vi "User Interface.vi"(8 "error in":errorcluster, 11 "User Interface in":refnum<class "User Interface.lvclass">=refnum) -> (0 "error out":errorcluster, 3 "User Interface out":refnum<class "User Interface.lvclass">)   [LabVIEW 2020, in "RDMA.lvlib" / "RDMA Transfer Tx User Interface.lvclass"]
uses:
  RDMA Transfer Tx User Interface.lvclass
  Configuration/Tx Transfer/RDMA Transfer Tx Configuration.lvclass
  DSF Core.lvlibp/Classes/User Interface/User Interface.lvclass
panel:
  in  "Local Port":u16
  in  "Local Address":string
  in  "Destination Address":string
  in  "Destination Port":u16
  # "RDMA Plugin Settings"
  # "* The address fields must be in IP dot notation. \n   Example: 10.0.53.23"
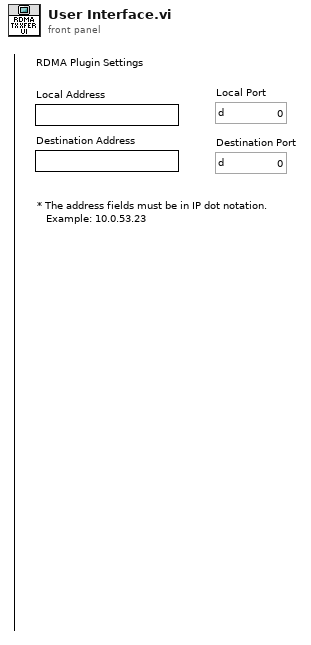
[diagram p1: front panel]
types:
  T1 = typedef "RDMA.lvlib/RDMA Transfer Tx Configuration.lvclass/Tx Transfer Settings.ctl" = cluster{"local address":u32, "local port":u16, "destination address":u32, "destination port":u16}
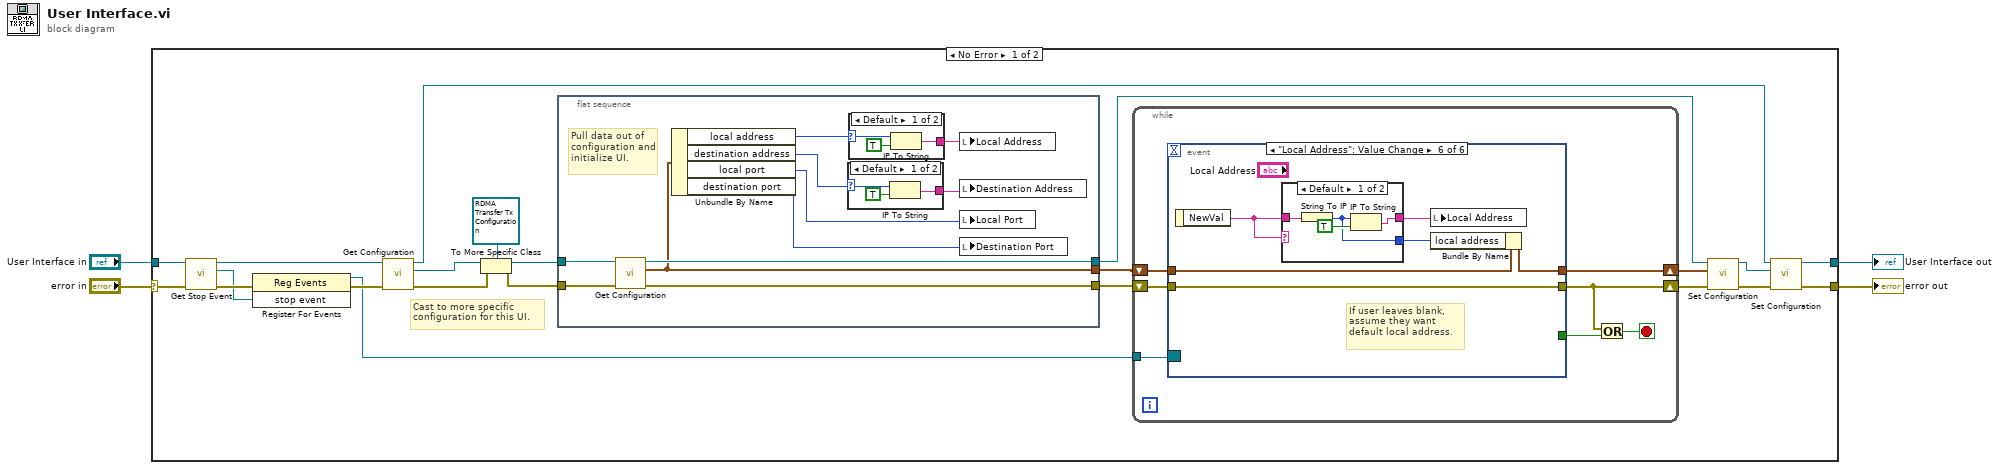
[diagram p0: block diagram]
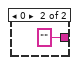
[diagram p2: hidden frame]
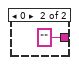
[diagram p3: hidden frame]
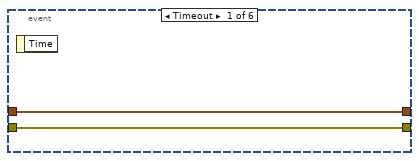
[diagram p4: hidden frame]
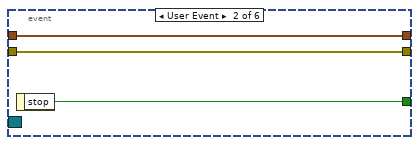
[diagram p5: hidden frame]
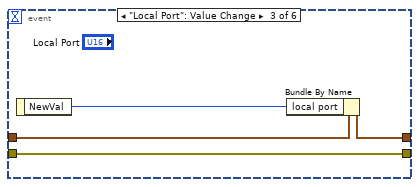
[diagram p6: hidden frame]
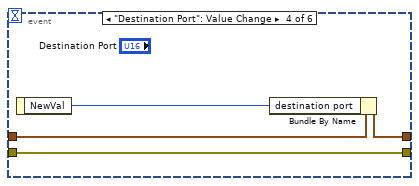
[diagram p7: hidden frame]
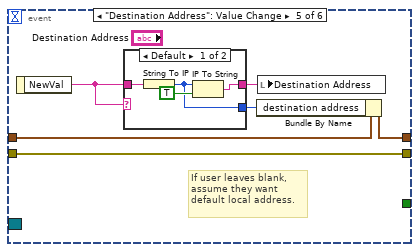
[diagram p8: hidden frame]
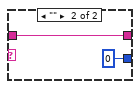
[diagram p9: hidden frame]
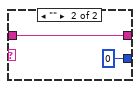
[diagram p10: hidden frame]
diagram:
  n1 = case shown="No Error" "error in" {
    selector: "error in" -> [w26 w91]
    tunnel: [w17 w91] -> w4
    tunnel: "User Interface in" -> [w25 w90]
    tunnel: [w16 w90] -> w1
    frame No Error {
      # "Cast to more specific configuration for this UI."
      n2 = call "Get Stop Event.vi"("error in (no error)"=w26, "User Interface in"=w25) -> ("error out"=w24:errorcluster, "stop event"=w23:refnum<user-event>, "User Interface out"=w22:refnum<class "User Interface.lvclass">)  [unwired: 7 in]
      n3 = register-events(error in=w24, w23) -> (reference out=w20:refnum<event-registration>, error out=w21:errorcluster)  [unwired: 1 in]
      n4 = call "Get Configuration.vi"("error in (no error)"=w21, "User Interface in"=w22) -> ("error out"=w19:errorcluster, "configuration"=w18:refnum<class "Configuration.lvclass">, "User Interface out"=w15:refnum<class "User Interface.lvclass">)  [unwired: 7 in]
      n5 = To More Specific Class(target class=refnum<class "RDMA Transfer Tx Configuration.lvclass"> refnum ("DSF Core.lvlib:UDP Transfer Tx Configuration.lvclass"), reference=w18, error in=w19) -> (specific class reference=w9:refnum<class "RDMA Transfer Tx Configuration.lvclass">, error out=w8:errorcluster)
      n6 = flat-sequence {
        tunnel: [w35] -> w5
        tunnel: w8 -> [w37]
        tunnel: w9 -> [w36]
        tunnel: [w33] -> w7
        tunnel: [w32] -> w6
        frame #0 {
          # "Pull data out of configuration and initialize UI."
          n7 = call "Get Configuration.vi"("error in"=w37, "RDMA Transfer Tx Configuration in"=w36) -> ("error out"=w35:errorcluster, "transfer settings"=w32:T1, "RDMA Transfer Tx Configuration out"=w33:refnum<class "RDMA Transfer Tx Configuration.lvclass">)  [unwired: 7 in]
          n8 = Unbundle By Name(w32) -> ("local address"=w31:u32, "destination address"=w30:u32, "local port"=w28:u16, "destination port"=w27:u16)
          n9 = case shown="Default" w30 {
            selector: w30 -> [w38 _]
            tunnel: [w40 "" ("name")] -> w29
            frame Default {
              n10 = IP To String(1:TRUE ("dot notation? (F)"), 2:w38) -> (0:w40:string)
            }
            frame 0 {
            }
          }
          n11 = case shown="Default" w31 {
            selector: w31 -> [w42 _]
            tunnel: [w44 "" ("name")] -> w34
            frame Default {
              n12 = IP To String(1:TRUE ("dot notation? (F)"), 2:w42) -> (0:w44:string)
            }
            frame 0 {
            }
          }
          n13 = local write "Local Address"(w34) -> ()
          n14 = local write "Destination Address"(w29) -> ()
          n15 = local write "Local Port"(w28) -> ()
          n16 = local write "Destination Port"(w27) -> ()
        }
      }
      n17 = while {
        tunnel: w20 -> [w49]
        shift-right: [w47] -> w13
        shift-left: w5 -> [w50]
        shift-right: [w46] -> w11
        shift-left: w6 -> [w51]
        stop <- w52 stop-if-true
        n18 = event shown="[5] \"Local Address\": Value Change" {
          selector: w49 -> [_ _ _ _ _ _]
          dyn-events: _ -> [_ _ _ _ _ _]
          timeout: _ -> [_ _ _ _ _ _]
          tunnel: [_ w56 _ _ _ _] -> w48
          tunnel: w50 -> [w54 w57 w61 w65 w68 w80]
          tunnel: [w54 w57 w61 w65 w68 w80] -> w47
          tunnel: w51 -> [w53 w55 w60 w64 w69 w81]
          tunnel: [w53 w55 w59 w63 w71 w83] -> w46
          event Timeout {
            n19 = event-data() -> ()  [unwired: 1 in, 1 out]
          }
          event User Event {
            n20 = event-data() -> ("stop"=w56:bool)  [unwired: 1 in]
          }
          event "Local Port": Value Change {
            n21 = event-data() -> ("NewVal"=w58:u16)  [unwired: 1 in]
            n22 = Bundle By Name(cluster=w60, "local port"=w58) -> (w59:T1)
          }
          event "Destination Port": Value Change {
            n23 = event-data() -> ("NewVal"=w62:u16)  [unwired: 1 in]
            n24 = Bundle By Name(cluster=w64, "destination port"=w62) -> (w63:T1)
          }
          event "Destination Address": Value Change {
            # "If user leaves blank, assume they want default local address."
            n25 = event-data() -> ("NewVal"=w66:string)  [unwired: 1 in]
            n26 = case shown="Default" w66 {
              tunnel: [w75 w76] -> w70
              tunnel: w66 -> [w74 w76]
              tunnel: [w72 u32 0] -> w67
              frame Default {
                n27 = String To IP(1:w74) -> (0:w72:u32)
                n28 = IP To String(1:TRUE ("dot notation? (F)"), 2:w72) -> (0:w75:string)
              }
              frame "" {
              }
            }
            n29 = Bundle By Name(cluster=w69, "destination address"=w67) -> (w71:T1)
            n30 = local write "Destination Address"(w70) -> ()
          }
          event "Local Address": Value Change {
            # "If user leaves blank, assume they want default local address."
            n31 = event-data() -> ("NewVal"=w78:string)  [unwired: 1 in]
            n32 = case shown="Default" w78 {
              tunnel: [w87 w88] -> w82
              tunnel: w78 -> [w86 w88]
              tunnel: [w84 u32 0] -> w79
              frame Default {
                n33 = String To IP(1:w86) -> (0:w84:u32)
                n34 = IP To String(1:TRUE ("dot notation? (F)"), 2:w84) -> (0:w87:string)
              }
              frame "" {
              }
            }
            n35 = local write "Local Address"(w82) -> ()
            n36 = Bundle By Name(cluster=w81, "local address"=w79) -> (w83:T1)
          }
        }
        n37 = Or(x=w47, y=w48) -> (x .or. y?=w52:bool)
      }
      n38 = call "Set Configuration.vi"("error in"=w13, "transfer settings"=w11, "RDMA Transfer Tx Configuration in"=w7) -> ("error out"=w12:errorcluster, "RDMA Transfer Tx Configuration out"=w10:refnum<class "RDMA Transfer Tx Configuration.lvclass">)  [unwired: 7 in]
      n39 = call "Set Configuration.vi"("error in (no error)"=w12, "configuration"=w10, "User Interface in"=w15) -> ("error out"=w17:errorcluster, "User Interface out"=w16:refnum<class "User Interface.lvclass">)  [unwired: 7 in]
    }
    frame Error {
    }
  }
  "error out" <- w4
  "User Interface out" <- w1
